vi "File_BrowseDirectoryRecursivly.vi"(0 "DirPath":path, 1 "Treat LLB as directories?":bool, 5 "error in (no error)":errorcluster, 6 "Reset":bool) -> (12 "Ctts":T1[](array[typedef]), 14 "VIs":T1[](array[typedef]), 15 "Ctls":T1[](array[typedef]), 16 "VITs":T1[](array[typedef]), 17 "All":T1[](array[typedef]), 19 "error out":errorcluster)   [LabVIEW 2020]
uses:
  File_FileInfo.ctl
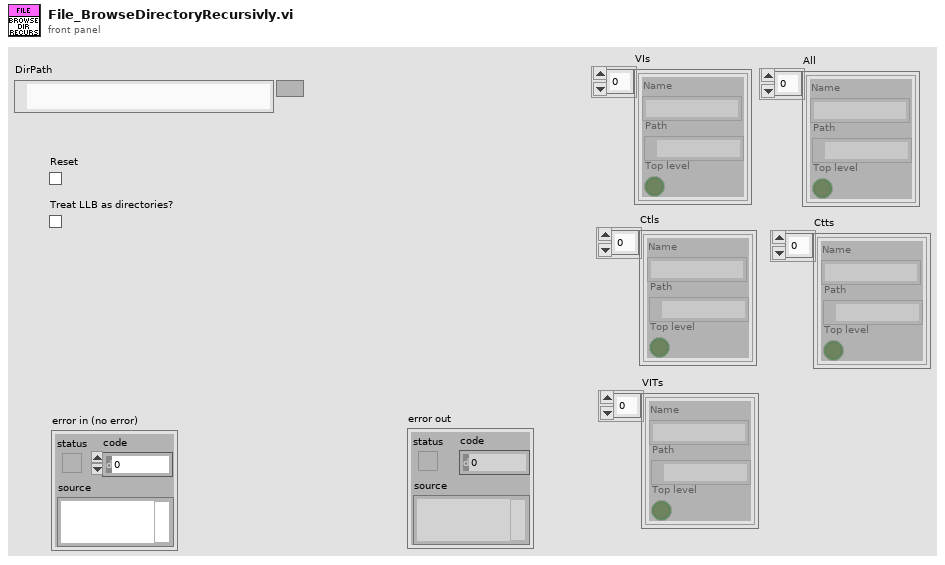
[diagram p1: front panel]
types:
  T1 = typedef "File_FileInfo.ctl" = cluster{"Name":string, "Path":path, "Top level":bool}
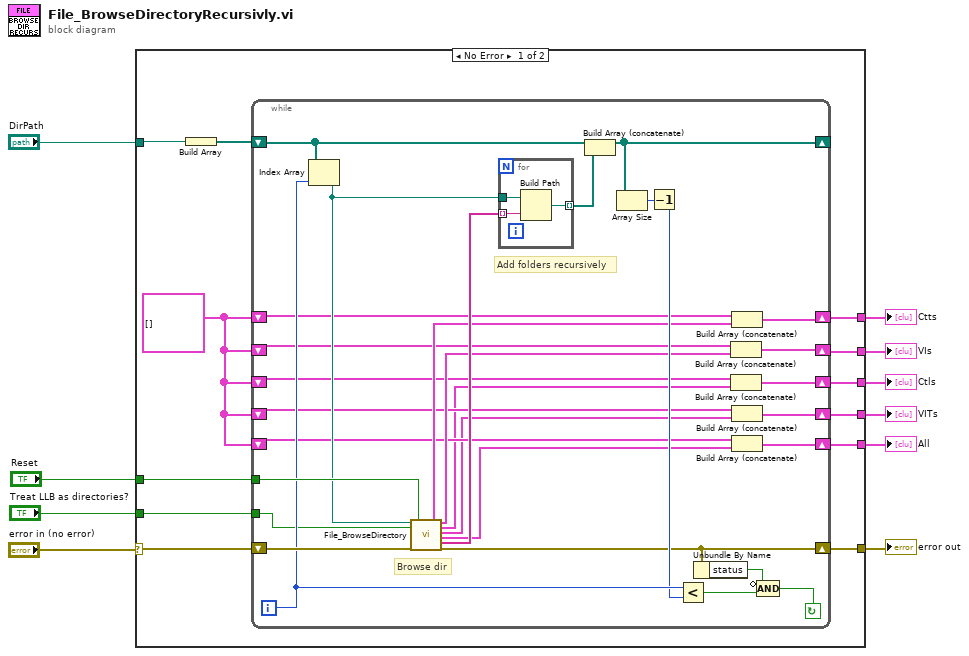
[diagram p0: block diagram]
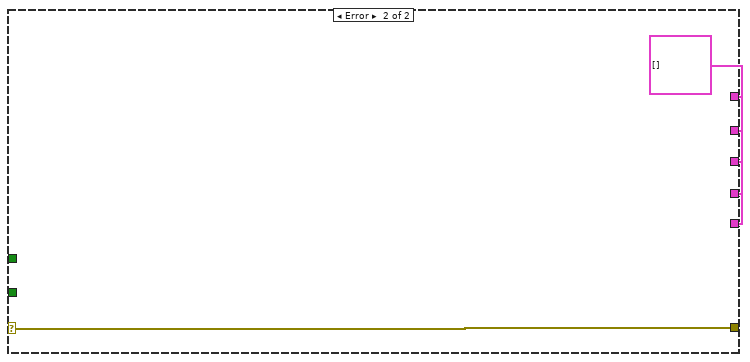
[diagram p2: hidden frame]
diagram:
  n1 = case shown="No Error" "error in (no error)" {
    selector: "error in (no error)" -> [w22 w57]
    tunnel: [w18 w57] -> w9
    tunnel: "DirPath" -> [w20 _]
    tunnel: "Reset" -> [w21 _]
    tunnel: [w16 w56] -> w6
    tunnel: [w15 w56] -> w5
    tunnel: [w14 w56] -> w4
    tunnel: [w13 w56] -> w3
    tunnel: [w12 w56] -> w2
    tunnel: "Treat LLB as directories?" -> [w11 _]
    frame No Error {
      w17 = T1[] [] ("Ctts")
      n2 = Build Array(w20) -> (w19:path[])
      n3 = while {
        tunnel: w11 -> [w23]
        shift-left: w17 -> [w27]
        shift-right: [w30] -> w16
        shift-left: w17 -> [w28]
        shift-right: [w31] -> w15
        shift-left: w17 -> [w29]
        shift-right: [w32] -> w14
        shift-left: w17 -> [w35]
        shift-right: [w33] -> w13
        shift-left: w17 -> [w38]
        shift-right: [w36] -> w12
        shift-left: w19 -> [w47]
        shift-right: [w46] -> _
        tunnel: w21 -> [w51]
        shift-left: w22 -> [w52]
        shift-right: [w41] -> w18
        i -> [w44]
        stop <- w39 continue-if-true
        # "Add folders recursively"
        # "Browse dir"
        n4 = Index Array(array=w47, index=w44) -> (element=w48:path)
        n5 = call "File_BrowseDirectory.vi"("DirPath"=w48, "Treat LLB as directories?"=w23, "error in (no error)"=w52, "Reset"=w51) -> ("Ctts"=w37:T1[], "VIs"=w34:T1[], "Ctls"=w26:T1[], "VITs"=w25:T1[], "All"=w24:T1[], "directory names"=w50:string[], "error out"=w41:errorcluster)  [unwired: 9 out]
        n6 = for {
          tunnel: w50 -> [w55] mode=indexing
          tunnel: w48 -> [w54]
          tunnel: [w53] -> w49 mode=indexing
          n7 = Build Path(base path=w54, name or relative path=w55) -> (appended path=w53:path)
        }
        n8 = Build Array (concatenate)(w47, w49) -> (w46:path[])
        n9 = Array Size(array=w46) -> (size(s)=w45:i32)
        n10 = Decrement(x=w45) -> (x-1=w43:i32)
        n11 = Less?(x=w44, y=w43) -> (x < y?=w42:bool)
        n12 = Unbundle By Name(w41) -> ("status"=w40:bool)
        n13 = Build Array (concatenate)(w35, w34) -> (w33:T1[])
        n14 = Build Array (concatenate)(w29, w26) -> (w32:T1[])
        n15 = Build Array (concatenate)(w38, w37) -> (w36:T1[])
        n16 = Build Array (concatenate)(w28, w25) -> (w31:T1[])
        n17 = Build Array (concatenate)(w27, w24) -> (w30:T1[])
        n18 = Compound Arithmetic op=AND(invert w40, w42) -> (w39:bool)
      }
    }
    frame Error {
      w56 = T1[] [] ("Ctts")
    }
  }
  "error out" <- w9
  "VITs" <- w5
  "Ctls" <- w4
  "VIs" <- w3
  "All" <- w6
  "Ctts" <- w2
